vi "Three Digit Nominal Vlaue Calculator.vi"(0 "1D sel":T2, 1 "2D sel":T2, 2 "3D sel":T2, 3 "M sel":T1) -> (6 "Nominal":dbl)   [LabVIEW 2018]
uses:
  digit--enum.ctl
  multiplier--enum.ctl
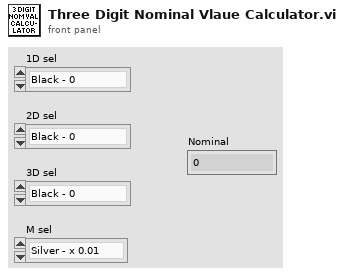
[diagram p1: front panel]
types:
  T1 = typedef "multiplier--enum.ctl" = enum16{"Silver - x 0.01", "Gold - x 0.1 ", "Black - x 1", "Brown - x 10", "Red - x 100", "Orange - x 1k", "Yellow - x 10k", "Green - 100k", "Blue - x 1M", "Violet - x10 M", "Grey - x 100M", "White - x 1G"}
  T2 = typedef "digit--enum.ctl" = enum16{"Black - 0", "Brown - 1", "Red - 2", "Orange - 3", "Yellow - 4", "Green - 5", "Blue - 6", "Violet - 7", "Grey - 8", "White - 9"}
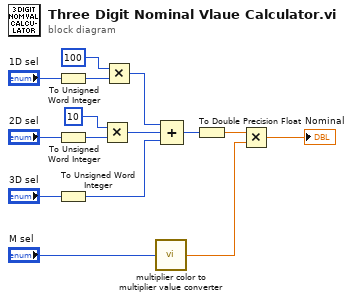
[diagram p0: block diagram]
diagram:
  n1 = To Unsigned Word Integer(number="1D sel") -> (unsigned 16bit integer=w1:u16)
  n2 = To Unsigned Word Integer(number="2D sel") -> (unsigned 16bit integer=w8:u16)
  n3 = To Unsigned Word Integer(number="3D sel") -> (unsigned 16bit integer=w14:u16)
  n4 = Multiply(x=u16 10, y=w8) -> (x*y=w9:u16)
  n5 = Multiply(x=u16 100 ("y"), y=w1) -> (x*y=w2:u16)
  n6 = call "multiplier color to multiplier value converter.vi"("mult color"="M sel") -> ("multiplier"=w6:dbl)  [unwired: 6 in]
  n7 = Compound Arithmetic op=ADD(w2, w9, w14) -> (w4:u16)
  n8 = To Double Precision Float(number=w4) -> (double precision float=w5:dbl)
  n9 = Multiply(x=w5, y=w6) -> (x*y=→"Nominal":dbl)
